vi "macro_NumCmd_Recv_OneDbl.vi"() -> ()   [LabVIEW 2019, in "Trajectory_Library.lvlib"]
uses:
  VI/BoolCmd_Recv_Internal.vi
  VI/BoolCmd_ObtainQueue.vi
  Trajectory_Library.lvlib
panel:
  out "ElevatorHeightDemand-Ft":dbl
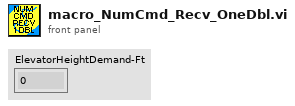
[diagram p1: front panel]
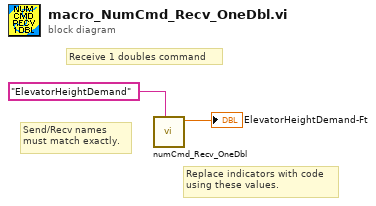
[diagram p0: block diagram]
diagram:
  # "Send/Recv names\nmust match exactly."
  # "Replace indicators with code\nusing these values."
  # "Receive 1 doubles command"
  n1 = call "numCmd_Recv_OneDbl.vi"("Command Name"="ElevatorHeightDemand") -> ("Value"=→"ElevatorHeightDemand-Ft":dbl)  [unwired: 8 in, 2 out]
